vi "Power_supply_keitley.vi"() -> ()   [LabVIEW 2017]
panel:
  out "XY Graph 2":cluster{dbl[], dbl[]}(graph)
  in  "I array":dbl[](array[numeric])
  in  "V array":dbl[](array[numeric])
  out "XY Graph":cluster{sgl[], sgl[]}(graph)
  out "P Chart 3":cluster{"Voltage":sgl, "Current":sgl}(graph)
  in  "VISA resource name":refnum<visa-resource-name>
  out "Power":sgl
  out "P Chart 2":sgl(graph)
  out "I Chart":sgl(graph)
  out "V Chart":sgl(graph)
  out "Current":sgl
  out "Voltage":sgl
  in  "Source Mode  (0: Voltage)":u16(ring) items=["Voltage", "Current"]
  in  "Compliance  Level (0.1)":dbl=0.1
  in  "Vini":dbl
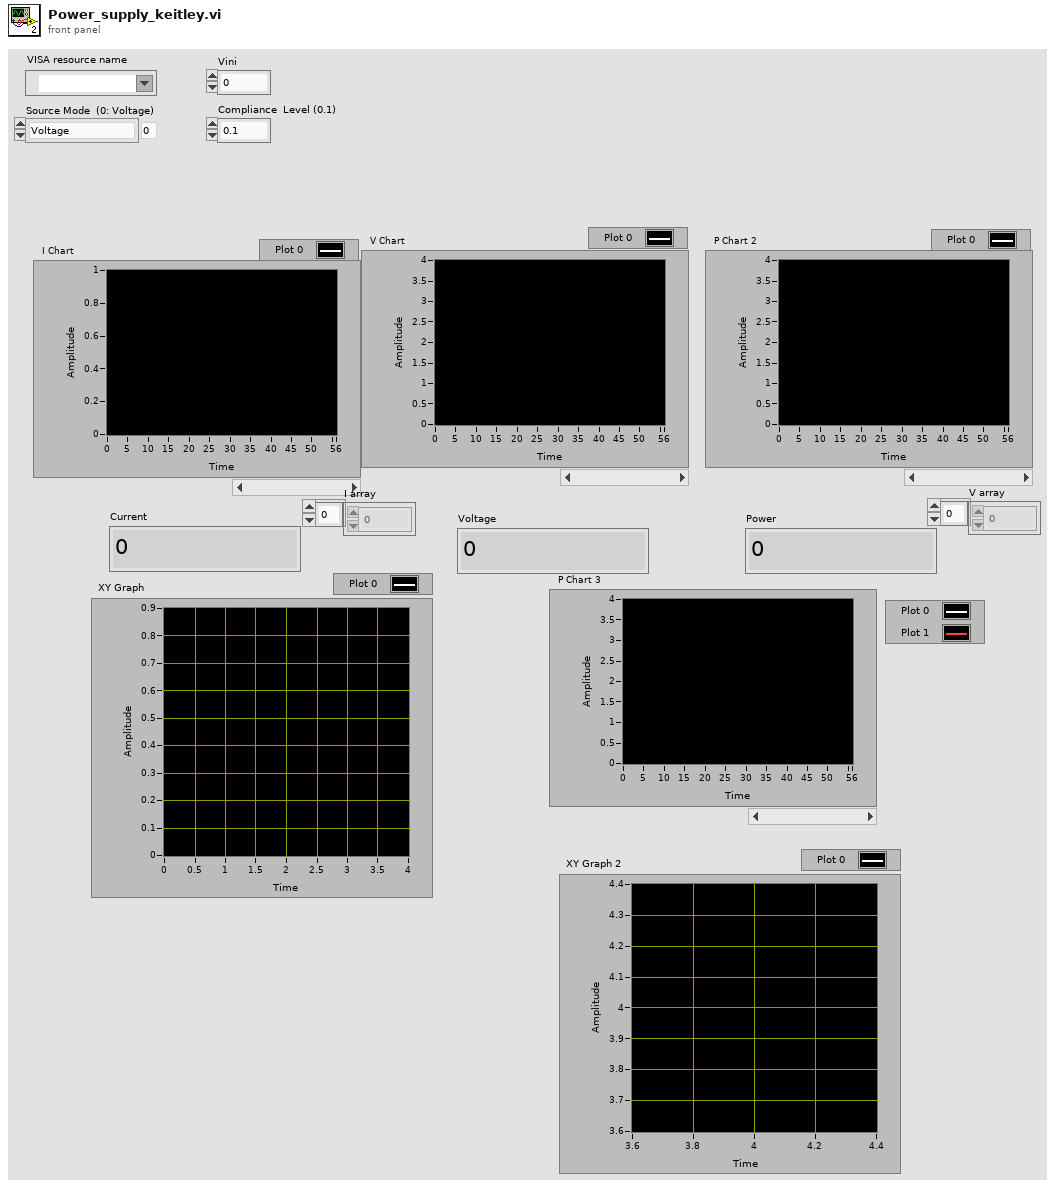
[diagram p1: front panel]
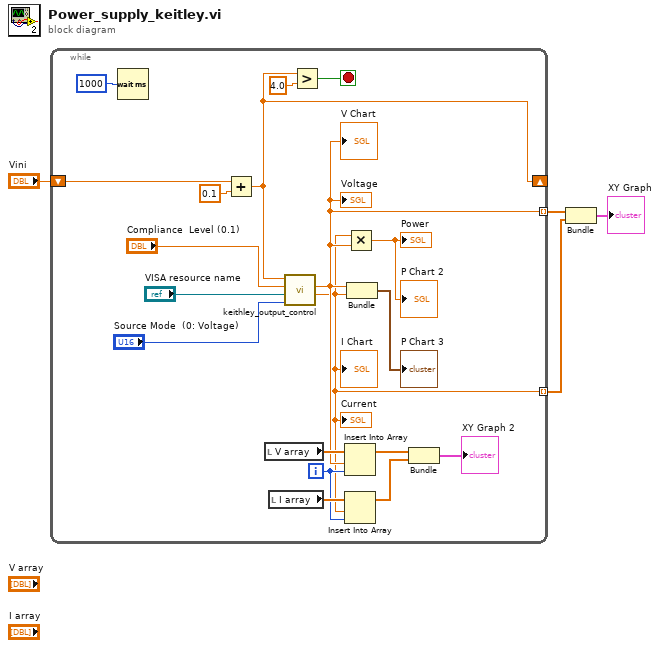
[diagram p0: block diagram]
diagram:
  n1 = while {
    shift-right: [w7] -> _
    shift-left: "Vini" -> [w20]
    tunnel: [w6] -> w3 mode=indexing
    tunnel: [w5] -> w2 mode=indexing
    i -> [w12]
    stop <- w21 stop-if-true
    n2 = Wait (ms)(milliseconds to wait=u32 1000) -> ()  [unwired: 1 out]
    n3 = Add(x=w20, y=0.1 ("x")) -> (x+y=w7:dbl)
    n4 = local read "V array"() -> (w17:dbl[])
    n5 = local read "I array"() -> (w16:dbl[])
    n6 = call "keithley_output_control.vi"("Source Mode  (0: Voltage)"="Source Mode  (0: Voltage)", "VISA resource name"="VISA resource name", "Compliance  Level (0.1)"="Compliance  Level (0.1)", "Output Level (0)"=w7) -> ("Current"=w5:sgl, "Voltage"=w6:sgl)  [unwired: 5 in, 1 out]
    "Voltage" <- w6
    "Current" <- w5
    "V Chart" <- w6
    "I Chart" <- w5
    n7 = Greater?(x=w7, y=4.0 ("x")) -> (0:w21:bool)
    n8 = Insert Into Array(array=w17, index=w6, new element=w12) -> (w15:dbl[])
    n9 = Insert Into Array(array=w16, index=w5, new element=w12) -> (w14:dbl[])
    n10 = Multiply(x=w5, y=w6) -> (x*y=→"P Chart 2" →"Power":sgl)
    n11 = Bundle("Voltage"=w6, "Current"=w5) -> (→"P Chart 3":cluster{"Voltage":sgl, "Current":sgl})  [unwired: 1 in]
    n12 = Bundle("V array"=w15, "I array"=w14) -> (→"XY Graph 2":cluster{"V array":dbl[], "I array ":dbl[]})  [unwired: 1 in]
  }
  n13 = Bundle(w3, w2) -> (→"XY Graph":cluster{sgl[], sgl[]})  [unwired: 1 in]
